vi "sortSeprateLayerImagesByAsendingHead.vi"(8 "error in (no error)":errorcluster, 10 "filenames":string[](array[string])=["20240925_DL2_s30_BlueGreen_DOE126_109-114-515-507_layer3_515.bmp", "20240925_DL2_s30_BlueGreen_DOE126_109-114-515-507_layer4_507.bmp", "20240925_DL2_s30_BlueGreen_DOE126_109-114-515-507_layer1_109.bmp", "20240925_DL2_s30_BlueGreen_DOE126_109-114-515-507_layer2_114.bmp"], 11 "Data Value Reference in":T1) -> (0 "error out":errorcluster, 1 "Materials":string[](array[string]), 2 "filenamesSortedbyAscndingHeads":string[](array[string]), 3 "Sorted Heads[]":u8[](array[numeric]))   [LabVIEW 2022 SP3, in "DLP2.lvclass"]
uses:
  DLP2.lvclass
  <vilib>/TELLC/Dynamic CVT API/TD Dynamic CVT DVR--ref.ctl
  Common/Controls/DLP_MaterialToHeadMapping--Cluster.ctl
  DataTypes/DLP2_PrinterMaterialProperties.ctl
  <userlib>/_OpenG.lib/array/array.llb/Sort 1D Array (U8)__ogtk.vi
  <userlib>/_OpenG.lib/array/array.llb/Index 1D Array Elements (String)__ogtk.vi
  DLP2.lvclass/DLP2.ctl
panel:
  out "Array 2":string[](array[string])
  out "Array":string[](array[string])
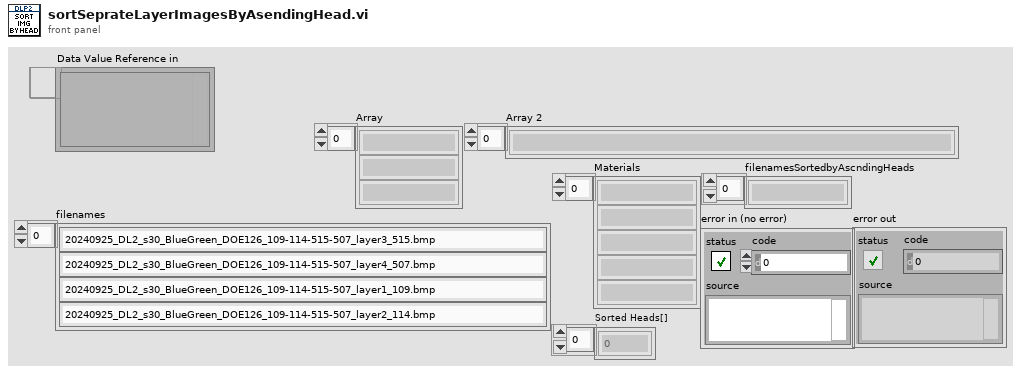
[diagram p1: front panel]
types:
  T1 = typedef "TD Dynamic CVT DVR--ref.ctl" = refnum<data-value>
  T2 = typedef "DLP_MaterialToHeadMapping--Cluster.ctl" = cluster{"Head":u8, "Ink":T3}
  T3 = typedef "DLP2_PrinterMaterialProperties.ctl" = cluster{"#attributes":cluster{"InkType":string, "PrePrintPurge":bool, "PurgeTime":dbl, "PurgeCount":i32, "Density":dbl, "NumberofDrops":i32, "PrintWeight":dbl, "PrintheadPrime":bool}, "Idle":cluster{"Name":string, "Heat":dbl, "Meniscus":dbl, "Recirculation":bool}[], "Process":cluster{"Name":string, "Heat":dbl, "Meniscus":dbl, "Recirculation":bool, "ColorPlane":string}[]}
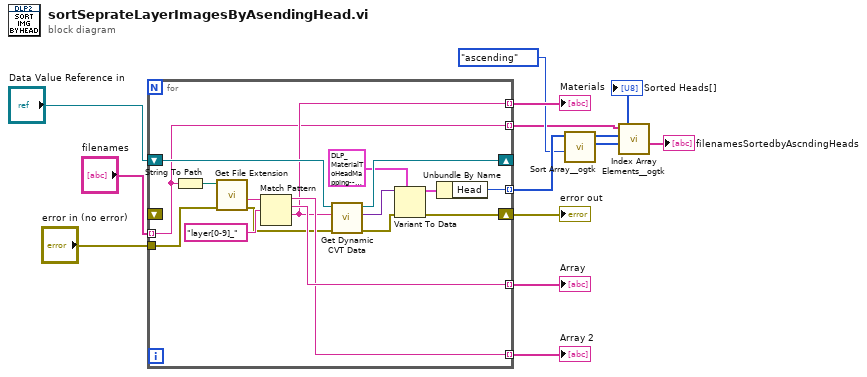
[diagram p0: block diagram]
diagram:
  n1 = for {
    tunnel: "filenames" -> [w18] mode=indexing
    shift-right: [w29] -> _
    shift-left: "Data Value Reference in" -> [w30]
    tunnel: [w28] -> w11 mode=indexing
    tunnel: [w27] -> w10 mode=indexing
    tunnel: [w23] -> w9 mode=indexing
    tunnel: [w19] -> w8 mode=indexing
    tunnel: [w18] -> w6 mode=indexing
    tunnel: "error in (no error)" -> [w15]
    shift-right: [w16] -> w2
    shift-left: _ -> [_]
    n2 = String To Path(string=w18) -> (path=w25:path)
    n3 = call <vilib>:"Get File Extension.vi"("error in (no error)"=w15, "file"=w25) -> ("error out"=w14:errorcluster, "filename without extension"=w24:string)  [unwired: 5 in, 3 out]
    n4 = Match Pattern(string=w24, regular expression="layer[0-9]_") -> (before substring=w27:string, match substring=w28:string, after substring=w23:string)  [unwired: 1 in, 1 out]
    n5 = call <vilib>:"Get Dynamic CVT Data.vi"("error in (no error)"=w14, "DataName"=w23, "dCVT DVR"=w30) -> ("error out"=w17:errorcluster, "value"=w22:variant, "dCVT DVR out"=w29:T1)  [unwired: 5 in, 1 out]
    n6 = Variant To Data(error in=w17, type=T2 {"Head"=0, "Ink"={"#attributes"={"InkType"="", "PrePrintPurge"=FALSE, "PurgeTime"=0.0, "PurgeCount"=0, "Density"=0.0, "NumberofDrops"=0, "PrintWeight"=0.0, "PrintheadPrime"=FALSE}, "Idle"=[], "Process"=[]}}, Variant=w22) -> (data=w20:T2, error out=w16:errorcluster)
    n7 = Unbundle By Name(w20) -> ("Head"=w19:u8)
  }
  "Array" <- w11
  "Array 2" <- w10
  "Materials" <- w9
  "error out" <- w2
  n8 = call-poly <userlib>:"Sort Array__ogtk.vi"("Order"=enum16{"ascending", "descending"}."ascending", "Array in"=w8) -> ("Sorted Pointers"=w5:i32[], "Sorted Array out"=→"Sorted Heads[]":u8[])  [unwired: 8 in]
  n9 = call-poly <userlib>:"Index Array Elements__ogtk.vi"("indices"=w5, "array"=w6) -> ("elements"=→"filenamesSortedbyAscndingHeads":string[])  [unwired: 9 in]
